vi "Pre-Init With Plugin.vi"(5 "REST Client in":refnum<class "REST Client.lvclass">, 8 "error in (no error)":errorcluster, 11 "http-client-type":refnum<class "Abstract HTTP Client.lvclass">) -> (0 "error out":errorcluster, 3 "REST Client out":refnum<class "REST Client.lvclass">)   [LabVIEW 2020, in "REST Client.lvlib" / "REST Client.lvclass"]
uses:
  REST Client.lvclass
  REST Client.lvclass/REST Client.ctl
  <vilib>/VIPM Community/HTTP Client Plugin - Base/Classes/Abstract HTTP Client/Abstract HTTP Client.lvclass
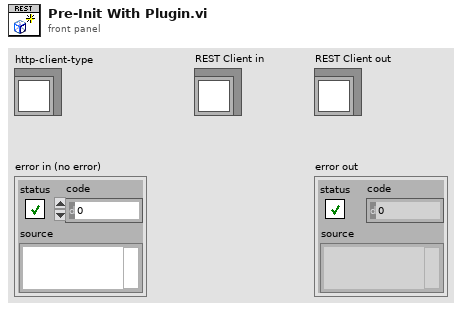
[diagram p1: front panel]
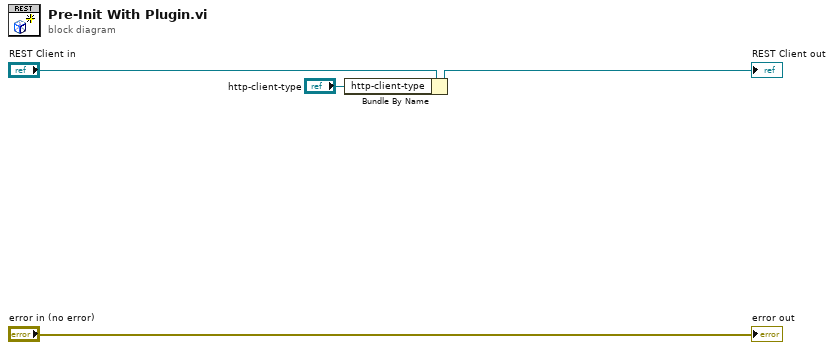
[diagram p0: block diagram]
diagram:
  n1 = Bundle By Name(cluster="REST Client in", "http-client-type"="http-client-type") -> (→"REST Client out":refnum<class "REST Client.lvclass">)
  "error out" <- "error in (no error)"
